vi "publisher tests Glue 5.vi"() -> ()   [LabVIEW 2018]
uses:
  publisher action.ctl
panel:
  out "request event":refnum<user-event>
  out "response event":refnum<user-event>
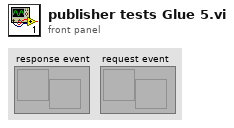
[diagram p1: front panel]
types:
  T1 = typedef "publisher action.ctl" = enum16{"set", "get", "init", "check"}
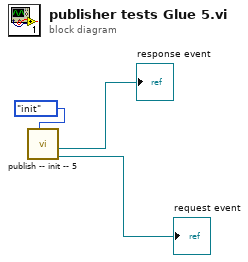
[diagram p0: block diagram]
diagram:
  n1 = call "publish -- init -- 5.vi"("publisher action"=publisher_action."init") -> ("request event"=→"request event":refnum<user-event>, "response event"=→"response event":refnum<user-event>)  [unwired: 9 in]
